vi "声发射频谱分析.vi"() -> ()   [LabVIEW 2014]
uses:
  <vilib>/Analysis/3filter.llb/Filter Passband Type.ctl
  <vilib>/Utility/error.llb/DialogType.ctl
  <vilib>/DAQmx/read.llb/DAQmx Read (Analog 1D Wfm NChan NSamp).vi
  <vilib>/DAQmx/create/channels.llb/DAQmx Create Channel (AI-Voltage-Basic).vi
  <vilib>/DAQmx/configure/timing.llb/DAQmx Timing (Sample Clock).vi
  <vilib>/DAQmx/miscellaneous.llb/DAQmx Fill In Error Info.vi
  <vilib>/Analysis/3filter.llb/Butterworth Filter (DBL).vi
  <vilib>/measure/mamon.llb/Waveform Peak Detection for 1 Chan.vi
  <vilib>/measure/maspectr.llb/FFT Power Spectral Density for 1 Chan.vi
  <vilib>/measure/maspectr.llb/FFT Spectrum (Mag-Phase) for 1 Chan.vi
  <vilib>/measure/NI_MAPro.lvlib
  <vilib>/Analysis/NI_AALBase.lvlib
panel:
  in  "stop":bool
  in  "high cutoff freq: fh":dbl=45.0 caption="高截止频率:fh" format="%0.2f"
  in  "low cutoff freq: fl":dbl=20000.0 caption="低截止频率:fl" format="%0.4f"
  in  "filter type":T1=enum."Highpass" caption="滤波器类型"
  in  "保存":bool
  in  "某通道 2":i32
  in  "Samples to Read":i32=100000 caption="读取采样数"
  in  "order":i32=8 caption="阶数"
  in  "Rate (Hz)":dbl=1000000.0 caption="采样率 (Hz)" format="%0.2f"
  in  "Physical Channel":tag="cDAQ9188-154541EMod1/ai1" caption="物理通道"
  in  "Minimum Value":dbl=-10.0 caption="最小值" format="%0.2f"
  in  "Maximum Value":dbl=10.0 caption="最大值" format="%0.2f"
  in  "选项卡控件":T2(tab)
  out "频域":cluster{"f0":dbl, "df":dbl, "magnitude":dbl[]}(graph)
  out "PSD":cluster{"f0":dbl, "df":dbl, "magnitude":dbl[]}(graph)
  out "Measurement 2":waveform(dbl)[](graph) caption="原始信号"
  out "Measurement":dbl[](graph) caption="滤波后信号"
  out "读取保存数据":waveform(dbl)(graph)
  out "振铃 2":i32[](graph)
  out "sum of Power spectral density 2":dbl[](graph)
  in  "End freq":dbl=200000.0
  in  "Start freq":dbl=20000.0
  out "sum of Power spectral density":dbl
  in  "阀值(volt)":dbl
  out "振铃":i32
  in  "某通道":i32
  out "大小":i32
  out "频域 2":cluster{"f0":dbl, "df":dbl, "magnitude":dbl[]}(graph)
  out "错误输出":errorcluster
  # "采集系统配置"
  # "系统操作"
  # "滤波"
  # "声发射信号采集分析"
  # "0.1 s"
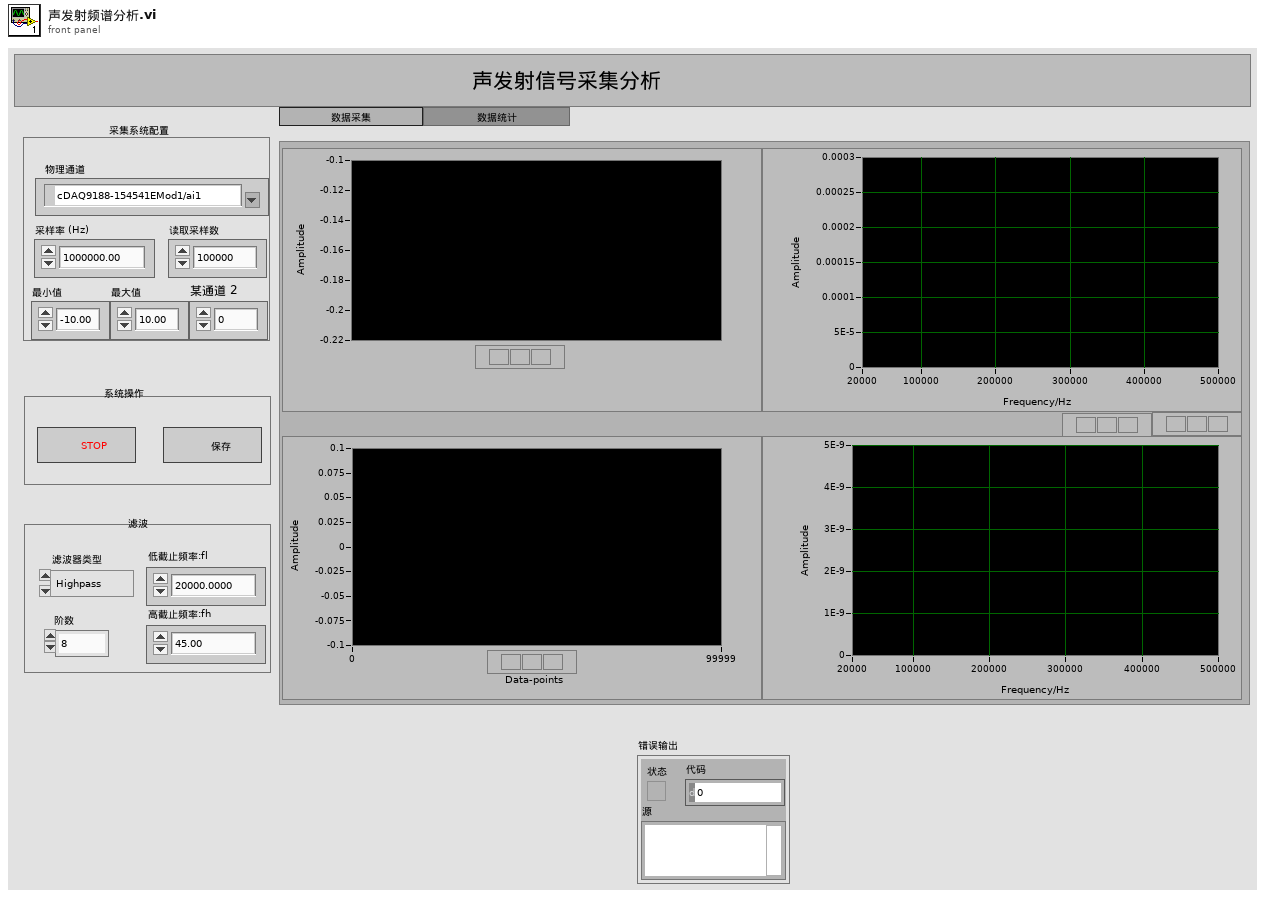
[diagram p1: front panel]
types:
  T1 = typedef "NI_AALBase.lvlib/Filter Passband Type.ctl" = enum32{"Lowpass", "Highpass", "Bandpass", "Bandstop"}
  T2 = enum32{"数据采集                              ", "数据统计                               "}
  T3 = enum16{"open", "open or create", "create or replace", "create", "open (read-only)"}
  T4 = typedef "DialogType.ctl" = u16
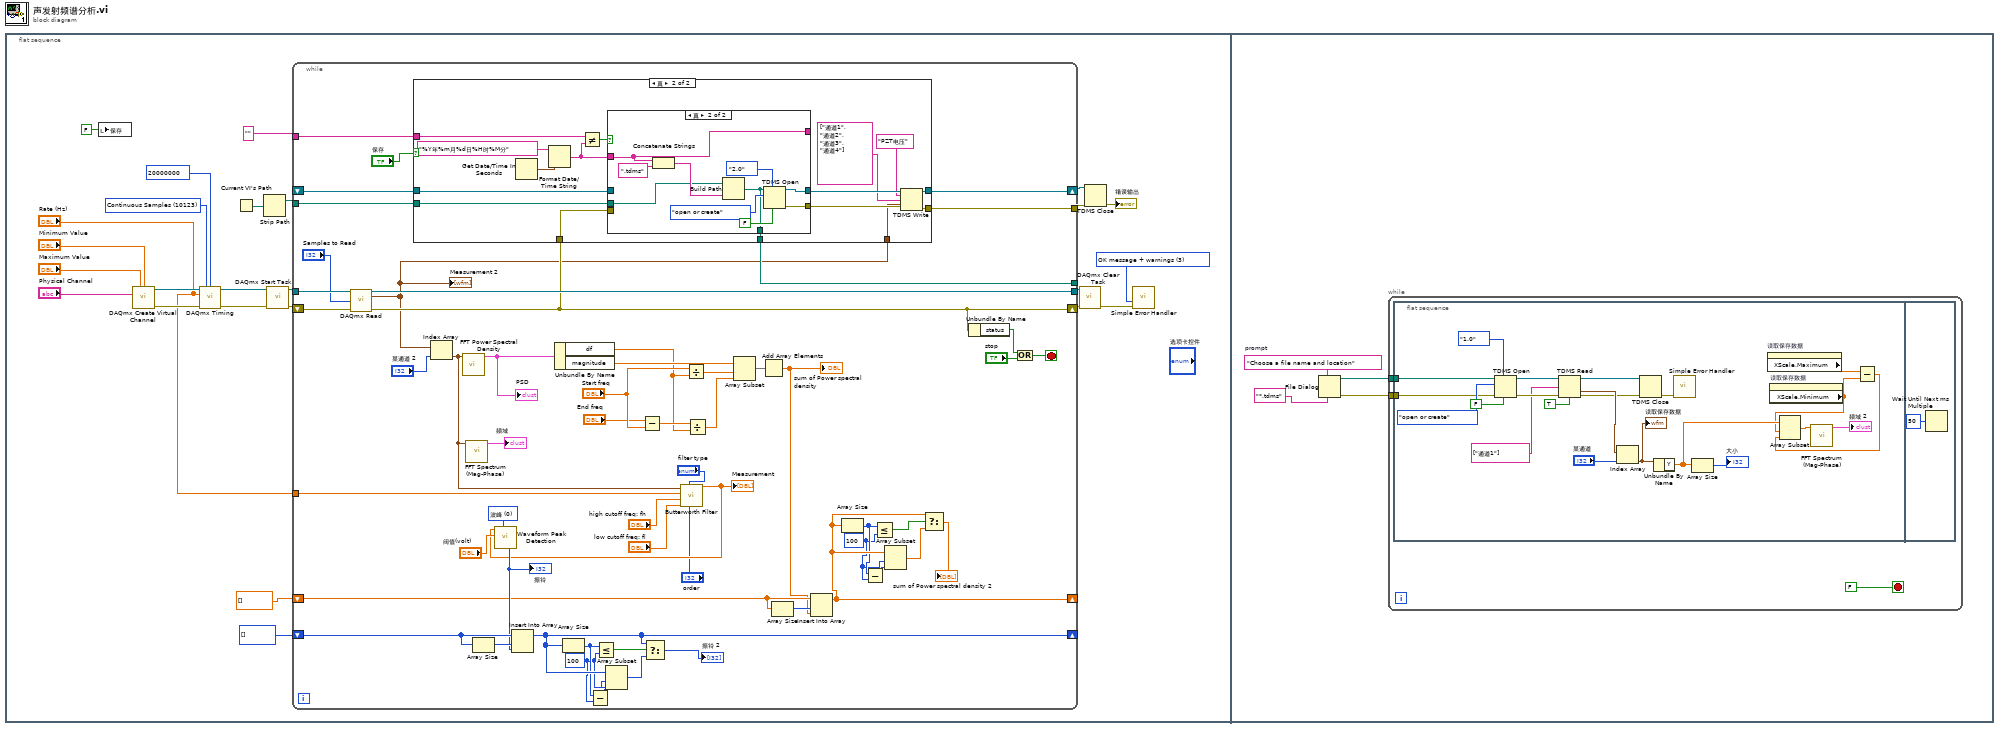
[diagram p0: block diagram]
diagram:
  n1 = flat-sequence {
    frame #0 {
      w15 = T4 3 items=["no dialog", "OK message", "continue or stop message", "OK message + warnings", "continue/stop + warnings"] ("type of dialog (OK msg:1)")
      w19 = 10123 items=["Finite Samples"=10178, "Continuous Samples"=10123, "Hardware Timed Single Point"=12522] ("sample mode")
      n2 = local write "保存"(FALSE ("保存")) -> ()
      n3 = call-poly <vilib>:"DAQmx Create Virtual Channel.vi"("maximum value"="Maximum Value", "minimum value"="Minimum Value", "physical channels"="Physical Channel") -> ("task out"=w23:refnum<k21>, "error out"=w20:errorcluster)  [unwired: 11 in]
      n4 = call-poly <vilib>:"DAQmx Timing.vi"("task/channels in"=w23, "sample mode"=w19, "samples per channel"=20000000 ("number of samples per channel"), "rate"="Rate (Hz)", "error in"=w20) -> ("task out"=w13:refnum<k21>, "error out"=w12:errorcluster)  [unwired: 9 in]
      n5 = Current VI's Path() -> (path=w11:path)
      n6 = Strip Path(path=w11) -> (stripped path=w9:path)  [unwired: 1 out]
      n7 = call <vilib>:"DAQmx Start Task.vi"("task/channels in"=w13, "error in"=w12) -> ("task out"=w25:refnum<k21>, "error out"=w21:errorcluster)  [unwired: 12 in]
      n8 = while {
        tunnel: w25 -> [w81]
        tunnel: [w80] -> w24
        shift-right: [w70] -> w22
        shift-left: w21 -> [w77]
        tunnel: "" ("子字符串") -> [w75]
        tunnel: w9 -> [w74]
        tunnel: [w72] -> w7
        shift-right: [w73] -> w8
        shift-left: _ -> [w71]
        tunnel: [w69] -> _
        shift-right: [w40] -> _
        shift-left: i32[] [] -> [w55]
        tunnel: "Rate (Hz)" -> [w52]
        shift-right: [w34] -> _
        shift-left: dbl[] [] -> [w45]
        stop <- w78 stop-if-true
        w27 = 100 ("# found")
        w31 = 100 ("# found")
        w56 = u16 0 items=["波峰", "波谷"] ("peaks/valleys")
        n9 = call-poly <vilib>:"DAQmx Read.vi"("task/channels in"=w81, "number of samples per channel"="Samples to Read", "error in"=w77) -> ("task out"=w80:refnum<k21>, "data"=w48:waveform(dbl)[], "error out"=w70:errorcluster)  [unwired: 10 in]
        "Measurement 2" <- w48
        n10 = case shown="真" "保存" {
          tunnel: w75 -> [_ w98]
          tunnel: w74 -> [w84 w97]
          tunnel: [w83 w92] -> w73
          tunnel: [w82 w91] -> w72
          tunnel: w71 -> [w83 w90]
          tunnel: w70 -> [w82 w89]
          tunnel: [w84 w87] -> w69
          tunnel: w48 -> [_ w85]
          frame False {
          }
          frame True {
            n11 = Get Date/Time In Seconds() -> (seconds since 1Jan1904=w99:timestamp)
            n12 = Format Date/Time String(time format string (%c)="%Y年%m月%d日%H时%M分" ("时间格式字符串(%c)"), seconds (now)=w99) -> (date/time string=w95:string)  [unwired: 1 in]
            n13 = Not Equal?(x=w98, y=w95) -> (x != y?=w96:bool)
            n14 = case shown="真" w96 {
              tunnel: w97 -> [w101 w109]
              tunnel: w95 -> [w103 w108]
              tunnel: [w103 w108] -> _
              tunnel: [w104 w107] -> w94
              tunnel: [w102 w106] -> w93
              tunnel: w90 -> [w104 _]
              tunnel: w89 -> [w102 _]
              tunnel: [w101 w105] -> w87
              frame False {
              }
              frame True {
                n15 = Concatenate Strings(w108, ".tdms" ("字符串")) -> (w114:string)
                n16 = Build Path(base path=w109, name or relative path=w114) -> (appended path=w105:path)
                n17 = TDMS Open(6:FALSE ("disable buffering (T)"), 7:enum16{"1.0", "2.0"}."2.0" ("file format version (2.0)"), 10:T3."open or create" ("operation"), 11:w105) -> (0:w106:errorcluster, 3:w107:refnum<k34>)  [unwired: 3 in]
              }
            }
            n18 = TDMS Write(0:w94, 5:"PZT电压" ("组名称输入（无标题）"), 7:string[] ["通道1", "通道2", "通道3", "通道4"] ("通道名输入（无标题）"), 9:w85, 11:w93) -> (4:w92:refnum<k34>, 15:w91:errorcluster)  [unwired: 1 in, 2 out]
          }
        }
        n19 = Index Array(array=w48, index="某通道 2") -> (element=w47:waveform(dbl))
        n20 = call-poly <vilib>:"FFT Power Spectral Density.vi"("time signal"=w47) -> ("power spectral density"=w60:cluster{"f0":dbl, "df":dbl, "magnitude":dbl[]})  [unwired: 7 in, 3 out]
        "PSD" <- w60
        n21 = call-poly <vilib>:"FFT Spectrum (Mag-Phase).vi"("time signal"=w47) -> ("magnitude"=→"频域":cluster{"f0":dbl, "df":dbl, "magnitude":dbl[]})  [unwired: 6 in, 4 out]
        n22 = Array Size(array=w55) -> (size(s)=w54:i32)
        n23 = Unbundle By Name(w60) -> ("df"=w59:dbl, "magnitude"=w62:dbl[])
        n24 = Subtract(x="End freq", y="Start freq") -> (x-y=w63:dbl)
        n25 = call-poly <vilib>:"Butterworth Filter.vi"("order"="order", "filter type"="filter type", "low cutoff freq: fl"="low cutoff freq: fl", "high cutoff freq: fh"="high cutoff freq: fh", "sampling freq: fs"=w52, "X"=w47) -> ("Filtered X"=w33:dbl[])  [unwired: 2 in, 1 out]
        "Measurement" <- w33
        n26 = call-poly <vilib>:"Waveform Peak Detection.vi"("peaks/valleys"=w56, "threshold"="阀值(volt)", "Signal In"=w33) -> ("# found"=w53:i32)  [unwired: 4 in, 4 out]
        "振铃" <- w53
        n27 = Insert Into Array(array=w55, index=w54, new element=w53) -> (w40:i32[])
        n28 = Array Size(array=w40) -> (size(s)=w32:i32)
        n29 = Subtract(x=w32, y=w31) -> (x-y=w30:i32)
        n30 = Less Or Equal?(x=w32, y=w31) -> (x <= y?=w41:bool)
        n31 = Array Subset(array=w40, index=w30, length=w31) -> (w38:i32[])
        n32 = Select(t=w40, s=w41, f=w38) -> (s? t:f=→"振铃 2":i32[])
        n33 = Divide(x="Start freq", y=w59) -> (x/y=w67:dbl)
        n34 = Divide(x=w63, y=w59) -> (x/y=w66:dbl)
        n35 = Array Subset(array=w62, index=w67, length=w66) -> (w68:dbl[])
        n36 = Add Array Elements(numeric array=w68) -> (sum=w44:dbl)
        "sum of Power spectral density" <- w44
        n37 = Array Size(array=w45) -> (size(s)=w46:i32)
        n38 = Insert Into Array(array=w45, index=w46, new element=w44) -> (w34:dbl[])
        n39 = Array Size(array=w34) -> (size(s)=w29:i32)
        n40 = Subtract(x=w29, y=w27) -> (x-y=w28:i32)
        n41 = Less Or Equal?(x=w29, y=w27) -> (x <= y?=w36:bool)
        n42 = Array Subset(array=w34, index=w28, length=w27) -> (w37:dbl[])
        n43 = Select(t=w34, s=w36, f=w37) -> (s? t:f=→"sum of Power spectral density 2":dbl[])
        n44 = Unbundle By Name(w70) -> ("status"=w79:bool)
        n45 = Or(x=w79, y="stop") -> (x .or. y?=w78:bool)
      }
      n46 = call <vilib>:"DAQmx Clear Task.vi"("task in"=w24, "error in"=w22) -> ("error out"=w14:errorcluster)  [unwired: 13 in]
      n47 = TDMS Close(8:w7, 11:w8) -> (0:→"错误输出":errorcluster)  [unwired: 1 out]
      n48 = call <vilib>:"Simple Error Handler.vi"("type of dialog (OK msg:1)"=w15, "error in (no error)"=w14) -> ()  [unwired: 3 in, 5 out]
    }
    frame #1 {
      w118 = "Choose a file name and location"  # prompt
      n49 = File Dialog(6:"*.tdms" ("pattern (all files)"), 7:w118) -> (0:w115:errorcluster, 3:w116:path)  [unwired: 1 in, 6 out]
      n50 = while {
        tunnel: w116 -> [w121]
        tunnel: w115 -> [w119]
        stop <- FALSE stop-if-true
        n51 = flat-sequence {
          tunnel: w119 -> [w124]
          tunnel: w121 -> [w135]
          frame #0 {
            n52 = TDMS Open(6:FALSE ("disable buffering (T)"), 7:enum16{"1.0", "2.0"}."1.0" ("file format version (2.0)"), 8:w124, 10:T3."open or create" ("operation"), 11:w135) -> (0:w132:errorcluster, 3:w133:refnum<k34>)  [unwired: 2 in]
            n53 = TDMS Read(0:w133, 7:string[] ["通道1"] ("通道名输入"), 11:w132, 13:TRUE ("return channels in file order? (F)")) -> (4:w136:refnum<k34>, 10:w125:waveform(dbl)[], 15:w123:errorcluster)  [unwired: 4 in, 3 out]
            n54 = Index Array(array=w125, index="某通道") -> (element=w122:waveform(dbl))
            "读取保存数据" <- w122
            n55 = TDMS Close(8:w123, 11:w136) -> (0:w137:errorcluster)  [unwired: 1 out]
            n56 = Unbundle By Name(w122) -> ("Y"=w143:dbl[])
            n57 = call <vilib>:"Simple Error Handler.vi"("error in (no error)"=w137) -> ()  [unwired: 1 in, 8 out]
            n58 = Array Size(array=w143) -> (size(s)=→"大小":i32)
            n59 = property on="读取保存数据" class="WFGraph (严格)"() -> ("XScale.Maximum"=w140:dbl)  [unwired: 2 in, 2 out]
            n60 = property on="读取保存数据" class="WFGraph (严格)"() -> ("XScale.Minimum"=w139:dbl)  [unwired: 2 in, 2 out]
            n61 = Subtract(x=w140, y=w139) -> (x-y=w138:dbl)
            n62 = Array Subset(array=w143, index=w139, length=w138) -> (w141:dbl[])
            n63 = call-poly <vilib>:"FFT Spectrum (Mag-Phase).vi"("time signal"=w141) -> ("magnitude"=→"频域 2":cluster{"f0":dbl, "df":dbl, "magnitude":dbl[]})  [unwired: 6 in, 4 out]
          }
          frame #1 {
            n64 = Wait Until Next ms Multiple(millisecond multiple=u32 50 ("毫秒倍数")) -> ()  [unwired: 1 out]
          }
        }
      }
    }
  }
